vi "MeasurementServer_Event_Close.vi"(0 "gRPCid":T1, 3 "error in (no error)":errorcluster) -> (10 "error out":errorcluster)   [LabVIEW 2019, in "labview-grpc-measurement-server.lvlib"]
uses:
  labview-grpc-measurement-server.lvlib
  MeasurementServer_gRPCid.ctl
  home/lvuser/liblabview_measurement_server.so
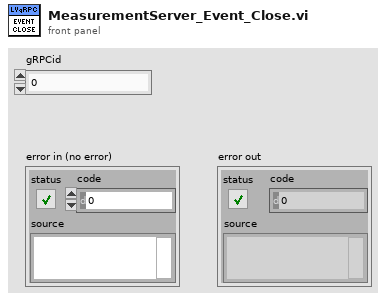
[diagram p1: front panel]
types:
  T1 = typedef "labview-grpc-measurement-server.lvlib/MeasurementServer_gRPCid.ctl" = u64
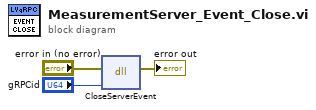
[diagram p0: block diagram]
diagram:
  n1 = dll-call lib="home/lvuser/liblabview_measurement_server.so" fn="CloseServerEvent"(error in="error in (no error)", "id"="gRPCid") -> (error out=→"error out":errorcluster)  [unwired: 4 in, 1 out]
